vi "Message from Header.vi"(8 "error in (no error)":errorcluster, 10 "Class name":string) -> (0 "error out":errorcluster, 3 "Serializable Msg out":refnum<class "Serializable Msg.lvclass">)   [LabVIEW 2020, in "Serializer.lvlib" / "Serializable Message.lvlib" / "Serializable Msg.lvclass"]
uses:
  Serializable Msg.lvclass
  App/Chat Window/Chat Window Messages/echo Msg/echo Msg.lvclass
  G:/Utilisateurs/hugofroylan.aragon/Documents/Nested Endpoint Actors Optimized/Serializer/Serializable Message/Serializable Msg.lvclass
  Serializable Msg.lvclass/Serializable Msg.ctl
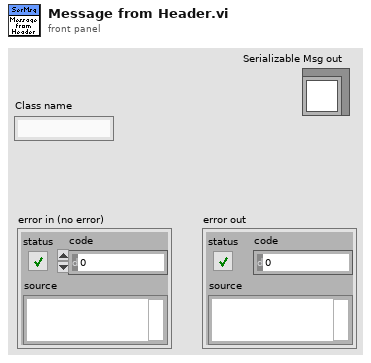
[diagram p1: front panel]
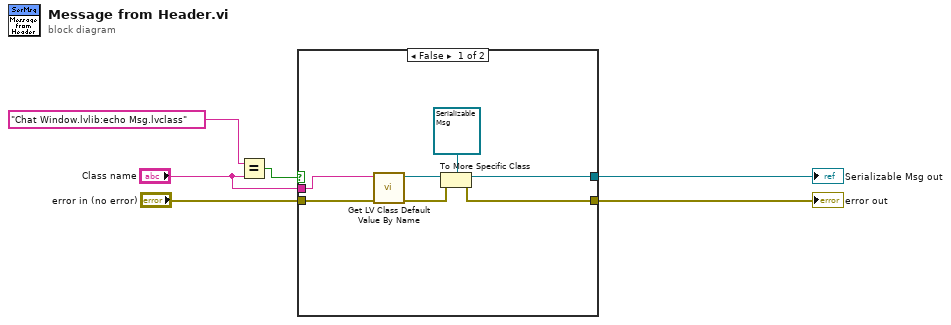
[diagram p0: block diagram]
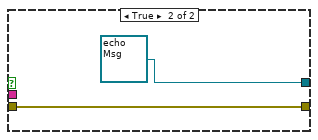
[diagram p2: hidden frame]
diagram:
  n1 = Equal?(x="Chat Window.lvlib:echo Msg.lvclass" ("class name"), y="Class name") -> (x = y?=w2:bool)
  n2 = case shown="False" w2 {
    tunnel: [w11 refnum<class "echo Msg.lvclass"> refnum ("Chat Window.lvlib:echo Msg.lvclass")] -> w6
    tunnel: [w10 w15] -> w5
    tunnel: "error in (no error)" -> [w8 w15]
    tunnel: "Class name" -> [w7 _]
    frame False {
      n3 = call <vilib>:"Get LV Class Default Value By Name.vi"("error in (no error)"=w8, "class name"=w7) -> ("error out"=w13:errorcluster, "object"=w9:refnum<class>)  [unwired: 8 in]
      n4 = To More Specific Class(target class=refnum<class "Serializable Msg.lvclass"> refnum ("Serializable Message.lvclass"), reference=w9, error in=w13) -> (specific class reference=w11:refnum<class "Serializable Msg.lvclass">, error out=w10:errorcluster)
    }
    frame True {
    }
  }
  "Serializable Msg out" <- w6
  "error out" <- w5
